vi "SnoSecondsForTraversal.vi"(0 "Volts Available":dbl format="%0.2f") -> (1 "Seconds for Traversal":dbl format="%0.2f", 2 "Interpolation Error":dbl format="%0.2f", 3 "In Range?":bool)   [LabVIEW 2014]
uses:
  <vilib>/Analysis/NI_AALPro.lvlib
panel:
  in  "Volts":dbl[](array[numeric])=[9.0, 10.0, 11.0, 12.0, 13.0, 14.0, 15.0] format="%0.2f"
  in  "Seconds":dbl[](array[numeric])=[1.0, 1.0, 1.0, 1.0, 1.0, 1.0, 1.0] format="%0.2f"
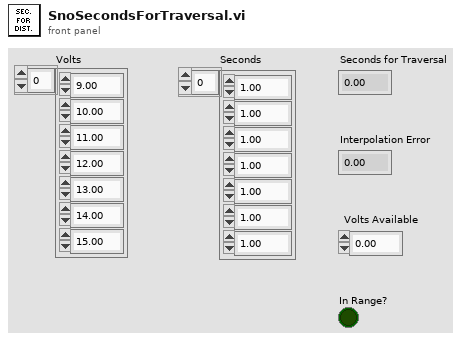
[diagram p1: front panel]
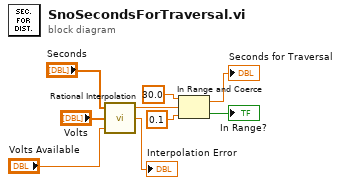
[diagram p0: block diagram]
diagram:
  n1 = call <vilib>:"Rational Interpolation.vi"("x value"="Volts Available", "X"="Volts", "Y"="Seconds") -> ("interpolation error"=→"Interpolation Error":dbl, "interpolation value"=w2:dbl)  [unwired: 1 out]
  n2 = In Range and Coerce(upper limit=30.0, x=w2, lower limit=0.1) -> (coerced(x)=→"Seconds for Traversal":dbl, In Range?=→"In Range?":bool)
